vi "Anritsu VNA Read Sweep Type.vi"(6 "Channel":i8=1 min=1 max=99 step=1, 7 "Anritsu VNA":T1, 8 "error in (no error)":errorcluster, 11 "VISA Resource Name":refnum<visa-resource-name>) -> (0 "error out":errorcluster, 2 "Sweep Type":T2, 3 "dup VISA Resource Name":refnum<visa-resource-name>)   [LabVIEW 2011]
doc: "This VI for the HP 8753 is used to read the sweep type.\n\n0 LINEAR FREQ\n1 LOG FREQ\n2 LIST FREQ\n3 CW TIME\n4 POWER SWEEP"
uses:
  TypeDefs/Anritsu VNA Sweep Type.ctl
  TypeDefs/Anritsu VNA Instrument Info.ctl
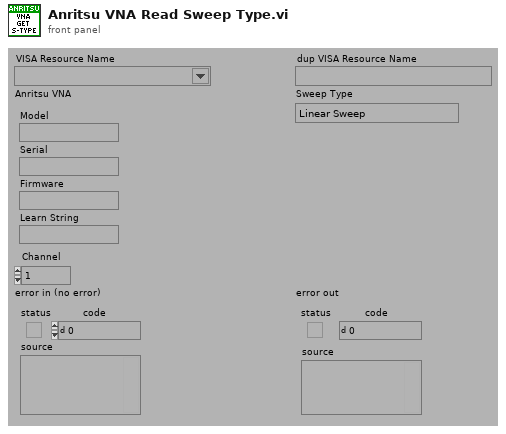
[diagram p1: front panel]
types:
  T1 = typedef "Anritsu VNA Instrument Info.ctl" = cluster{"Model":string, "Serial":string, "Firmware":string, "Learn String":string}
  T2 = typedef "Anritsu VNA Sweep Type.ctl" = enum32{"Linear Sweep", "Frequency Sweep", "Power Sweep", "CW Time Sweep", "Discrete Fill", "Time Domain", "Logarithmic Sweep", "Segmented Sweep (Frequency)", "Segmented Sweep (Index)", "MFGC"}
  T3 = typedef "Anritsu VNA Model.ctl" = enum16{"Not Supported", "37XXXX", "MS20XXX", "MS462XX", "MS464XX"}
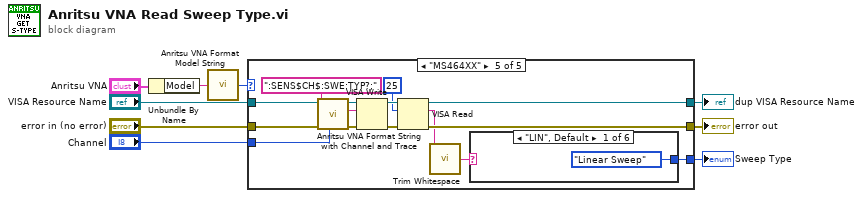
[diagram p0: block diagram]
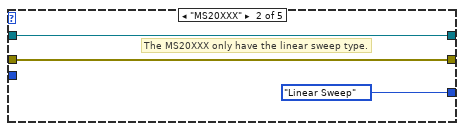
[diagram p3: hidden frame]
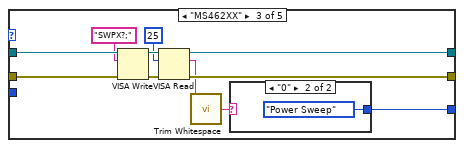
[diagram p4: hidden frame]
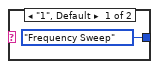
[diagram p5: hidden frame]
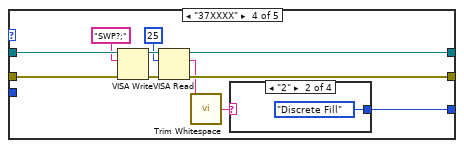
[diagram p6: hidden frame]
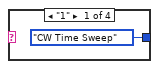
[diagram p7: hidden frame]
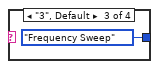
[diagram p8: hidden frame]
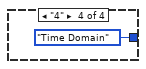
[diagram p9: hidden frame]
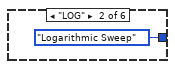
[diagram p10: hidden frame]
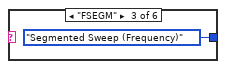
[diagram p11: hidden frame]
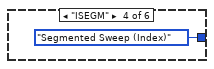
[diagram p12: hidden frame]
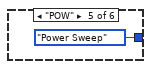
[diagram p13: hidden frame]
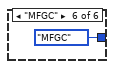
[diagram p14: hidden frame]
diagram:
  n1 = Unbundle By Name("Anritsu VNA") -> ("Model"=w3:string)
  n2 = call "Anritsu VNA Format Model String.vi"("Model"=w3) -> ("Model"=w2:T3)
  n3 = case shown="\"MS464XX\"" w2 {
    tunnel: "VISA Resource Name" -> [w10 w12 w22 w35 w52]
    tunnel: "error in (no error)" -> [w11 w13 w25 w38 w55]
    tunnel: [w11 w13 w20 w33 w50] -> w8
    tunnel: [_ Anritsu_VNA_Sweep_Type."Linear Sweep" ("sweep type") w18 w31 w49] -> w7
    tunnel: [w10 w12 w21 w34 w51] -> w5
    tunnel: "Channel" -> [_ _ _ _ w43]
    frame "Not Supported" {
    }
    frame "MS20XXX" {
      # "The MS20XXX only have the linear sweep type."
    }
    frame "MS462XX" {
      n4 = VISA Write(VISA resource name=w22, write buffer="SWPX?;", error in (no error)=w25) -> (VISA resource name out=w23:refnum<visa-resource-name>, error out=w24:errorcluster)  [unwired: 1 out]
      n5 = VISA Read(VISA resource name=w23, byte count=u32 25, error in (no error)=w24) -> (VISA resource name out=w21:refnum<visa-resource-name>, read buffer=w16:string, error out=w20:errorcluster)  [unwired: 1 out]
      n6 = call <vilib>:"Trim Whitespace.vi"("string"=w16) -> ("trimmed string"=w15:string)  [unwired: 1 in]
      n7 = case shown="\"0\"" w15 {
        tunnel: [Anritsu_VNA_Sweep_Type."Frequency Sweep" ("sweep type") Anritsu_VNA_Sweep_Type."Power Sweep" ("sweep type")] -> w18
        frame "1", Default {
        }
        frame "0" {
        }
      }
    }
    frame "37XXXX" {
      n8 = VISA Write(VISA resource name=w35, write buffer="SWP?;", error in (no error)=w38) -> (VISA resource name out=w36:refnum<visa-resource-name>, error out=w37:errorcluster)  [unwired: 1 out]
      n9 = VISA Read(VISA resource name=w36, byte count=u32 25, error in (no error)=w37) -> (VISA resource name out=w34:refnum<visa-resource-name>, read buffer=w29:string, error out=w33:errorcluster)  [unwired: 1 out]
      n10 = call <vilib>:"Trim Whitespace.vi"("string"=w29) -> ("trimmed string"=w28:string)  [unwired: 1 in]
      n11 = case shown="\"2\"" w28 {
        tunnel: [Anritsu_VNA_Sweep_Type."CW Time Sweep" ("sweep type") Anritsu_VNA_Sweep_Type."Discrete Fill" ("sweep type") Anritsu_VNA_Sweep_Type."Frequency Sweep" ("sweep type") Anritsu_VNA_Sweep_Type."Time Domain" ("sweep type")] -> w31
        frame "1" {
        }
        frame "2" {
        }
        frame "3", Default {
        }
        frame "4" {
        }
      }
    }
    frame "MS464XX" {
      n12 = call "Anritsu VNA Format String with Channel and Trace.vi"("Channel"=w43, "String"=":SENS$CH$:SWE:TYP?;" ("write buffer")) -> ("String Out"=w44:string)  [unwired: 1 in, 6 out]
      n13 = VISA Write(VISA resource name=w52, write buffer=w44, error in (no error)=w55) -> (VISA resource name out=w53:refnum<visa-resource-name>, error out=w54:errorcluster)  [unwired: 1 out]
      n14 = VISA Read(VISA resource name=w53, byte count=u32 25, error in (no error)=w54) -> (VISA resource name out=w51:refnum<visa-resource-name>, read buffer=w47:string, error out=w50:errorcluster)  [unwired: 1 out]
      n15 = call <vilib>:"Trim Whitespace.vi"("string"=w47) -> ("trimmed string"=w46:string)  [unwired: 1 in]
      n16 = case shown="\"LIN\", Default" w46 {
        tunnel: [Anritsu_VNA_Sweep_Type."Linear Sweep" ("sweep type") Anritsu_VNA_Sweep_Type."Logarithmic Sweep" ("sweep type") Anritsu_VNA_Sweep_Type."Segmented Sweep (Frequency)" ("sweep type") Anritsu_VNA_Sweep_Type."Segmented Sweep (Index)" ("sweep type") Anritsu_VNA_Sweep_Type."Power Sweep" ("sweep type") Anritsu_VNA_Sweep_Type."MFGC" ("sweep type")] -> w49
        frame "LIN", Default {
        }
        frame "LOG" {
        }
        frame "FSEGM" {
        }
        frame "ISEGM" {
        }
        frame "POW" {
        }
        frame "MFGC" {
        }
      }
    }
  }
  "Sweep Type" <- w7
  "dup VISA Resource Name" <- w5
  "error out" <- w8
